vi "SetPositionCOM.vi"(8 "error in":errorcluster, 9 "Axis":enum16{"X", "Y", "Z"}(ring), 10 "Position (mm)":dbl, 11 "VISA resource name":refnum<visa-resource-name>) -> (0 "error out":errorcluster, 3 "VISA resource name out":refnum<visa-resource-name>)   [LabVIEW 2017]
panel:
  out "Raw write string (hex)":string
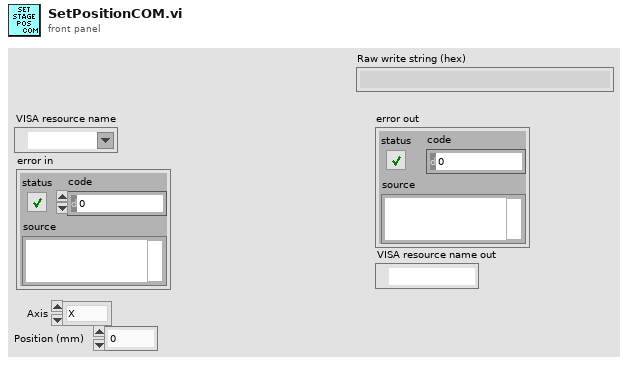
[diagram p1: front panel]
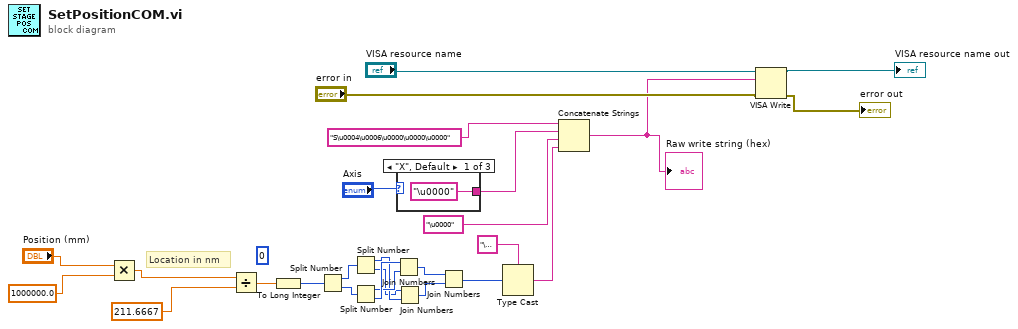
[diagram p0: block diagram]
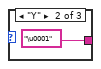
[diagram p2: hidden frame]
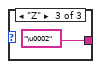
[diagram p3: hidden frame]
diagram:
  (unwired) 0 ("byte count")
  # "Location in nm"
  n1 = Multiply(x="Position (mm)", y=1000000.0) -> (x*y=w21:dbl)
  n2 = Divide(x=w21, y=211.6667) -> (x/y=w8:dbl)
  n3 = To Long Integer(number=w8) -> (32bit integer=w9:i32)
  n4 = Split Number(x=w9) -> (hi(x)=w19:u16, lo(x)=w18:u16)
  n5 = Split Number(x=w19) -> (hi(x)=w15:u8, lo(x)=w14:u8)
  n6 = Split Number(x=w18) -> (hi(x)=w16:u8, lo(x)=w17:u8)
  n7 = Join Numbers(hi=w17, lo=w16) -> ((hi.lo)=w12:u16)
  n8 = Join Numbers(hi=w14, lo=w15) -> ((hi.lo)=w13:u16)
  n9 = case shown="\"X\", Default" "Axis" {
    tunnel: ["\u0000" "\u0001" "\u0002"] -> w24
    frame "X", Default {
    }
    frame "Y" {
    }
    frame "Z" {
    }
  }
  n10 = Join Numbers(hi=w12, lo=w13) -> ((hi.lo)=w11:u32)
  n11 = Type Cast(type="\u0000", x=w11) -> (*(type *) &x=w2:string)
  n12 = Concatenate Strings("S\u0004\u0006\u0000\u0000\u0000", w24, "\u0000", w2) -> (w3:string)
  "Raw write string (hex)" <- w3
  n13 = VISA Write(VISA resource name="VISA resource name", write buffer=w3, error in (no error)="error in") -> (VISA resource name out=→"VISA resource name out":refnum<visa-resource-name>, error out=→"error out":errorcluster)  [unwired: 1 out]
